vi "Autonomous Independent.vi"() -> ()   [LabVIEW 2015]
doc: "This VI is called when autonomous begins, and will automatically be terminated when autonomous ends. You can carry out timed or sensor driven robot movement independently without needing to return to the caller."
uses:
  <vilib>/Rock Robotics/WPI/Utilities/WPI_GetSetVariantRefNum.vi
  <vilib>/Rock Robotics/Network Tables/NT Read String.vi
  <vilib>/Rock Robotics/WPI/RobotDrive/WPI_RobotDriveArcadeDrive_Standard(NoSaturation).vi
  <vilib>/Rock Robotics/Network Tables/NT Write Numeric Array.vi
  Robot Global Data.vi
  <vilib>/Rock Robotics/Network Tables/NT Read Number.vi
  <vilib>/Rock Robotics/WPI/Solenoid/WPI_SolenoidSetEnum.vi
  <vilib>/Rock Robotics/WPI/Solenoid/WPI_SolenoidValue.ctl
  <vilib>/Rock Robotics/WPI/Relay/WPI_RelayValue.ctl
panel:
  out "Current Movement, for debugging":T1 {"Y Joystick Value" scale=1.0..-1.0; "X Joystick Value" scale=-1.0..1.0}
  in  "Array of robot movements":T2(array[cluster])=[{"X Joystick Value"=0.39393939393939403, "Y Joystick Value"=0.0, "Delay (sec)"=1.0, "Movement Name"="turn"}, {"X Joystick Value"=-0.3737373737373737, "Y Joystick Value"=0.0, "Delay (sec)"=1.0, "Movement Name"="turn back"}] {"Y Joystick Value" scale=1.0..-1.0; "X Joystick Value" scale=-1.0..1.0}
  # "Be sure to right-click and choose Data Operations>>Make Current Value default if you want to save the array values with the VI"
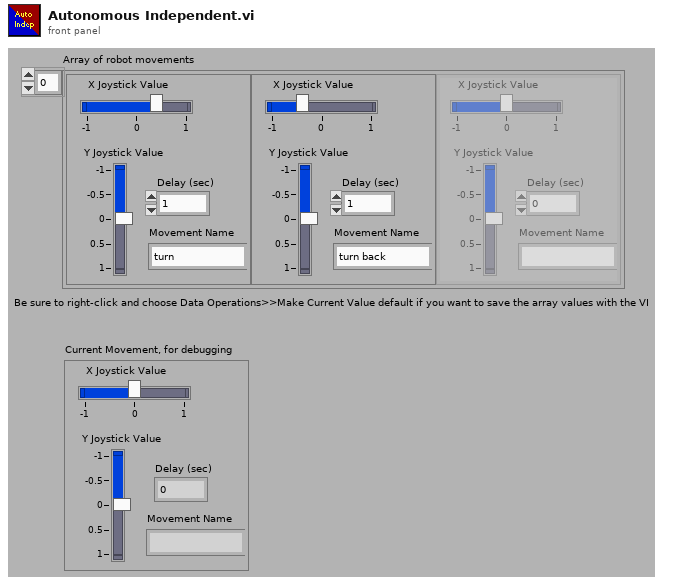
[diagram p1: front panel]
types:
  T1 = cluster{"X Joystick Value":dbl, "Y Joystick Value":dbl, "Delay (sec)":dbl, "Movement Name":string}
  T2 = cluster{"X Joystick Value":dbl, "Y Joystick Value":dbl, "Delay (sec)":dbl, "Movement Name":string}[]
  T3 = typedef "WPI_JoystickDevRef.ctl" = cluster{"Device":T4}
  T4 = typedef "WPI_JoystickDeviceEnum.ctl" = enum16{"USB 0", "USB 1", "USB 2", "USB 3", "USB 4", "USB 5"}
  T5 = typedef "WPI_RelayValue.ctl" = enum16{"Off", "On", "Forward", "Reverse"}
  T6 = typedef "WPI_SolenoidValue.ctl" = enum16{"Off", "On", "Forward", "Reverse"}
  T7 = typedef "WPI_RobotDriveDevRef.ctl" = cluster{"DevStatus":errorcluster, "Motors[]":T8[], "Square Inputs":bool, "Max Output":dbl}
  T8 = typedef "WPI_MotorControlDeviceRef.ctl" = cluster{"DeviceStatus":errorcluster, "Type":T9, "PWM":cluster{"PWM Channel":T10, "DeadBand":T11}, "CAN":cluster{"Device Number":u8, "Control Mode":T12, "Semaphore":T13, "Max Vout":dbl, "TalonSRX Control Mode":T14}, "Invert":bool}
  T9 = typedef "WPI_MotorControlType.ctl" = enum16{"PWM", "CAN", "CANTalonSRX"}
  T10 = typedef "FPGA_DIOPWMChannel.ctl" = enum8{"PWM 0", "PWM 1", "PWM 2", "PWM 3", "PWM 4", "PWM 5", "PWM 6", "PWM 7", "PWM 8", "PWM 9", "PWM MXP 0", "PWM MXP 1", "PWM MXP 2", "PWM MXP 3", "PWM MXP 4", "PWM MXP 5", "PWM MXP 6", "PWM MXP 7", "PWM MXP 8", "PWM MXP 9", "Invalid"}
  T11 = typedef "WPI_PWMDeadband.ctl" = cluster{"Name":string, "maxPositivePwm":i32, "minPositivePwm":i32, "centerPwm":i32, "maxNegativePwm":i32, "minNegativePwm":i32, "angularRange":u16}
  T12 = typedef "WPI_CANJaguar_ControlMode.ctl" = enum8{"Percent VBus", "Current", "Speed", "Position", "Voltage"}
  T13 = typedef "Semaphore RefNum" = refnum<k1>
  T14 = typedef "WPI_CANTalonSRX_APIControlMode.ctl" = enum8{"Percent VBus", "Speed", "Position", "Slave", "Unchanged / Invalid", "Voltage Compensation", "Current", "Motion Profile"}
  T15 = typedef "WPI_RelayDevRef.ctl" = cluster{"DevStatus":errorcluster, "Relay Channel":T16, "Relay Direction":T17}
  T16 = typedef "FPGA_DIORelayChannel.ctl" = enum8{"Relay 0", "Relay 1", "Relay 2", "Relay 3", "Invalid"}
  T17 = typedef "WPI_RelayDirection.ctl" = enum16{"Both directions", "Forward only", "Reverse only"}
  T18 = typedef "WPI_SolenoidDevRef.ctl" = cluster{"DevStatus":errorcluster, "Pneumatics Control Module":u8, "Forward Solenoid Channel":T19, "Reverse Solenoid Channel":T19}
  T19 = typedef "WPI_SolenoidChannel.ctl" = enum8{"Solenoid 0", "Solenoid 1", "Solenoid 2", "Solenoid 3", "Solenoid 4", "Solenoid 5", "Solenoid 6", "Solenoid 7", "Invalid"}
  T20 = cluster{"Distance (ft)":dbl, "Center":cluster{dbl, dbl}, "Normalized Rect":cluster{"Numeric":dbl, "Numeric 2":dbl, "Numeric 3":dbl, "Numeric 5":dbl}}[]
  T21 = cluster{"Distance (ft)":dbl, "Center":cluster{dbl, dbl}, "Normalized Rect":cluster{"Numeric":dbl, "Numeric 2":dbl, "Numeric 3":dbl, "Numeric 5":dbl}}
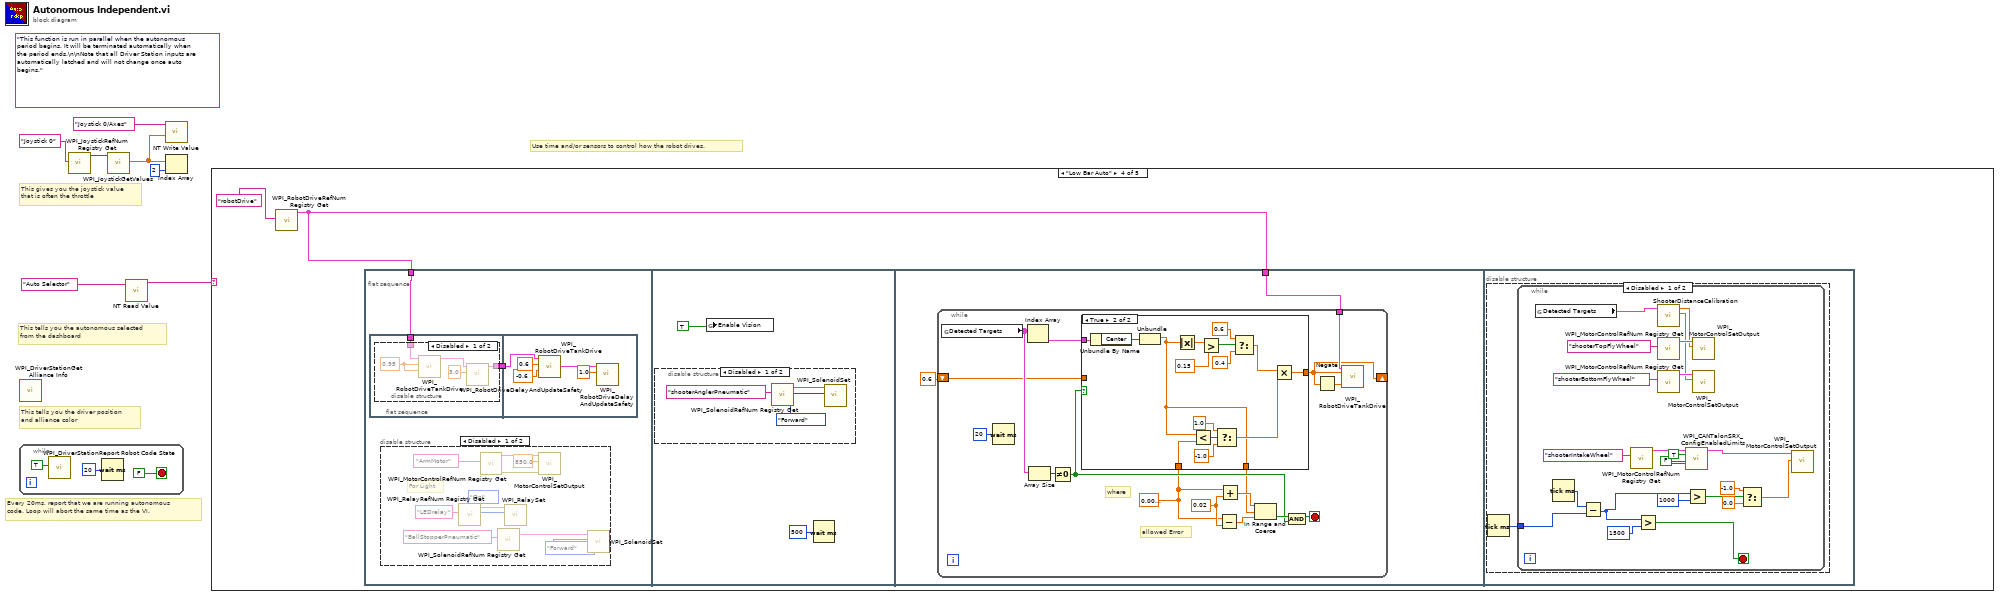
[diagram p0: block diagram]
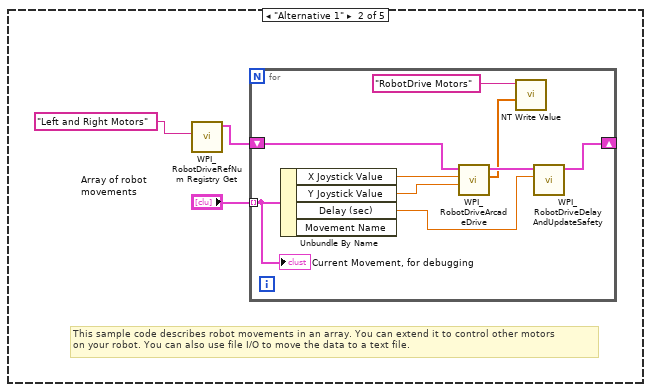
[diagram p3: hidden frame]
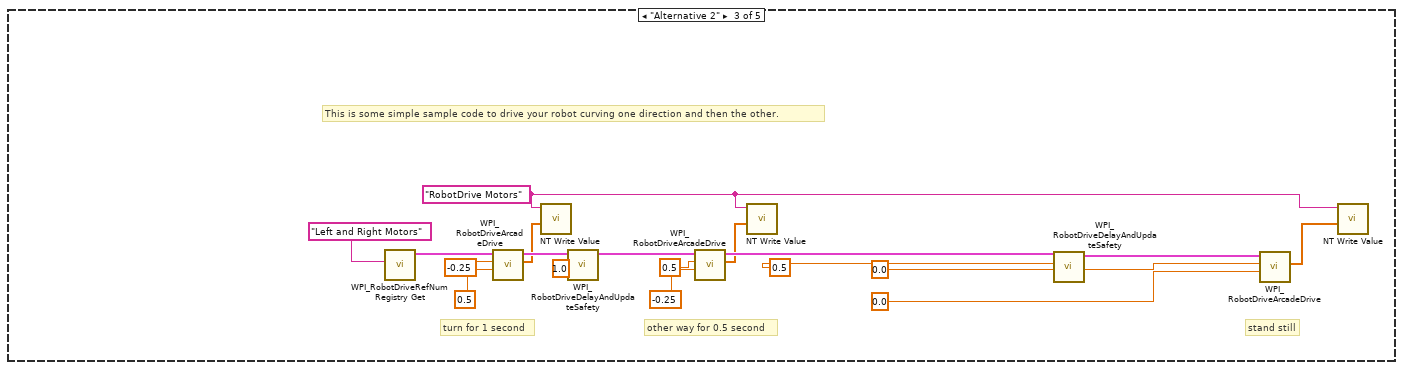
[diagram p4: hidden frame]
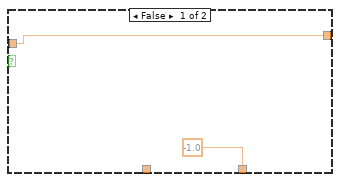
[diagram p8: hidden frame]
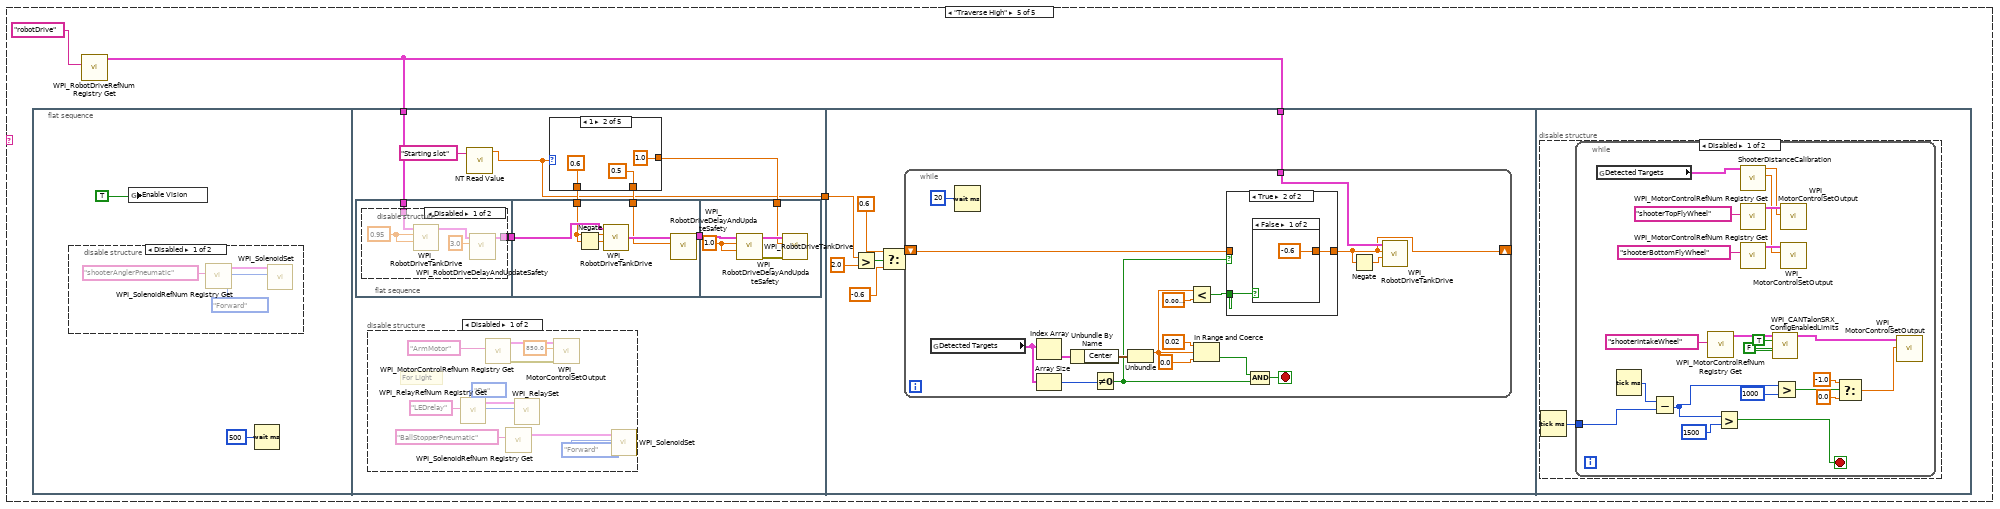
[diagram p10: hidden frame]
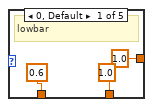
[diagram p12: hidden frame]
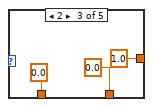
[diagram p13: hidden frame]
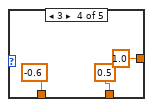
[diagram p14: hidden frame]
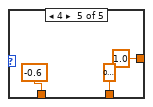
[diagram p15: hidden frame]
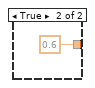
[diagram p19: hidden frame]
diagram:
  (unwired) "This function is run in parallel when the autonomous period begins. It will be terminated automatically when the period ends.\n\nNote that all Driver Station inputs are automatically latched and will not change once auto begins."
  # "This tells you the autonomous selected\nfrom the dashboard"
  # "Every 20ms, report that we are running autonomous\ncode. Loop will abort the same time as the VI."
  # "This gives you the joystick value\nthat is often the throttle"
  # "Use time and/or sensors to control how the robot drives."
  # "This tells you the driver position\nand alliance color"
  n1 = while {
    stop <- FALSE stop-if-true
    n2 = call <vilib>:"WPI_DriverStationReport Robot Code State.vi"("Autonomous"=TRUE) -> ()  [unwired: 10 in, 1 out]
    n3 = Wait (ms)(milliseconds to wait=u32 20) -> ()  [unwired: 1 out]
  }
  n4 = call <vilib>:"WPI_DriverStationGet Alliance Info.vi"() -> ()  [unwired: 12 out]
  n5 = call <vilib>:"WPI_JoystickRefNum Registry Get.vi"("refnum name"="Joystick 0") -> ("JoystickDevRef"=w6:T3)  [unwired: 1 in, 9 out]
  n6 = call <vilib>:"WPI_JoystickGetValues.vi"("JoystickDevRef"=w6) -> ("Axes"=w3:dbl[])  [unwired: 6 in, 4 out]
  n7 = call-poly <vilib>:"NT Read Value.vi"("Name"="Auto Selector") -> ("String"=w1:string)  [unwired: 9 in, 1 out]
  n8 = call-poly <vilib>:"NT Write Value.vi"("Numeric Array"=w3, "Name"="Joystick 0/Axes") -> ()  [unwired: 9 in, 1 out]
  n9 = Index Array(array=w3, index=2) -> ()  [unwired: 1 out]
  n10 = case shown="\"Low Bar Auto\"" w1 {
    frame "Nothing", Default {
      # "You can put your main auto here, or you can right-click on the case and make any\nother frame be the default case."
      # "This is the frame that will execute if no selection is made, or if it is not recognized"
    }
    frame "Alternative 1" {
      # "This sample code describes robot movements in an array. You can extend it to control other motors\non your robot. You can also use file I/O to move the data to a text file."
      n11 = call <vilib>:"WPI_RobotDriveRefNum Registry Get.vi"("refnum name"="Left and Right Motors") -> ("RobotDriveDevRef"=w12:T7)  [unwired: 1 in, 9 out]
      n12 = for {
        shift-right: [w20] -> _
        shift-left: w12 -> [w21]
        tunnel: "Array of robot movements" -> [w16] mode=indexing
        n13 = Unbundle By Name(w16) -> ("X Joystick Value"=w19:dbl, "Y Joystick Value"=w18:dbl, "Delay (sec)"=w17:dbl)  [unwired: 1 out]
        n14 = call-poly <vilib>:"WPI_RobotDriveArcadeDrive.vi"("Y axis value"=w18, "X axis value"=w19, "RobotDriveDevRef"=w21) -> ("Motor Values"=w14:dbl[], "RobotDriveDevRef"=w22:T7)  [unwired: 1 in, 6 out]
        n15 = call-poly <vilib>:"NT Write Value.vi"("Numeric Array"=w14, "Name"="RobotDrive Motors") -> ()  [unwired: 9 in, 1 out]
        n16 = call <vilib>:"WPI_RobotDriveDelayAndUpdateSafety.vi"("Delay (s)"=w17, "RobotDriveDevRef"=w22) -> ("RobotDriveDevRef 2"=w20:T7)  [unwired: 8 in, 1 out]
        "Current Movement, for debugging" <- w16
      }
    }
    frame "Alternative 2" {
      w24 = "RobotDrive Motors" ("Name")
      # "This is some simple sample code to drive your robot curving one direction and then the other."
      # "stand still"
      # "other way for 0.5 second"
      # "turn for 1 second"
      n17 = call <vilib>:"WPI_RobotDriveRefNum Registry Get.vi"("refnum name"="Left and Right Motors") -> ("RobotDriveDevRef"=w40:T7)  [unwired: 1 in, 9 out]
      n18 = call-poly <vilib>:"WPI_RobotDriveArcadeDrive.vi"("Y axis value"=0.5 ("X axis value"), "X axis value"=-0.25, "RobotDriveDevRef"=w40) -> ("Motor Values"=w23:dbl[], "RobotDriveDevRef"=w33:T7)  [unwired: 1 in, 6 out]
      n19 = call-poly <vilib>:"NT Write Value.vi"("Numeric Array"=w23, "Name"=w24) -> ()  [unwired: 9 in, 1 out]
      n20 = call <vilib>:"WPI_RobotDriveDelayAndUpdateSafety.vi"("Delay (s)"=1.0, "RobotDriveDevRef"=w33) -> ("RobotDriveDevRef 2"=w34:T7)  [unwired: 8 in, 1 out]
      n21 = call-poly <vilib>:"WPI_RobotDriveArcadeDrive.vi"("Y axis value"=-0.25 ("X axis value"), "X axis value"=0.5, "RobotDriveDevRef"=w34) -> ("Motor Values"=w25:dbl[], "RobotDriveDevRef"=w35:T7)  [unwired: 1 in, 6 out]
      n22 = call-poly <vilib>:"NT Write Value.vi"("Numeric Array"=w25, "Name"=w24) -> ()  [unwired: 9 in, 1 out]
      n23 = call <vilib>:"WPI_RobotDriveDelayAndUpdateSafety.vi"("Delay (s)"=0.5, "RobotDriveDevRef"=w35) -> ("RobotDriveDevRef 2"=w36:T7)  [unwired: 8 in, 1 out]
      n24 = call-poly <vilib>:"WPI_RobotDriveArcadeDrive.vi"("Y axis value"=0.0 ("X axis value"), "X axis value"=0.0, "RobotDriveDevRef"=w36) -> ("Motor Values"=w26:dbl[])  [unwired: 1 in, 7 out]
      n25 = call-poly <vilib>:"NT Write Value.vi"("Numeric Array"=w26, "Name"=w24) -> ()  [unwired: 9 in, 1 out]
    }
    frame "Low Bar Auto" {
      n26 = call <vilib>:"WPI_RobotDriveRefNum Registry Get.vi"("refnum name"="robotDrive") -> ("RobotDriveDevRef"=w41:T7)  [unwired: 9 in, 1 out]
      n27 = flat-sequence {
        tunnel: w41 -> [w44]
        tunnel: w41 -> [w73]
        frame #0 {
          n28 = flat-sequence {
            tunnel: w44 -> [w56]
            tunnel: [w55] -> w43
            tunnel: w43 -> [w63]
            frame #0 {
              n29 = disable-structure shown="Disabled" {
                disable-tunnel: w56 -> [w59 w62]
                disable-tunnel: [w58 w62] -> w55
                frame Disabled {
                  w57 = 0.95 ("Left axis value")
                  n30 = call <vilib>:"WPI_RobotDriveTankDrive.vi"("Right axis value"=w57, "Left axis value"=w57, "RobotDriveDevRef"=w59) -> ("RobotDriveDevRef"=w60:T7)  [unwired: 6 in, 2 out]
                  n31 = call <vilib>:"WPI_RobotDriveDelayAndUpdateSafety.vi"("Delay (s)"=3.0, "RobotDriveDevRef"=w60) -> ("RobotDriveDevRef 2"=w58:T7)  [unwired: 8 in, 1 out]
                }
                frame Enabled {
                }
              }
            }
            frame #1 {
              n32 = call <vilib>:"WPI_RobotDriveTankDrive.vi"("Right axis value"=-0.6, "Left axis value"=0.6, "RobotDriveDevRef"=w63) -> ("RobotDriveDevRef"=w66:T7)  [unwired: 6 in, 2 out]
              n33 = call <vilib>:"WPI_RobotDriveDelayAndUpdateSafety.vi"("Delay (s)"=1.0, "RobotDriveDevRef"=w66) -> ()  [unwired: 8 in, 2 out]
            }
          }
          n34 = disable-structure shown="Disabled" {
            frame Disabled {
              # "For Light"
              n35 = call <vilib>:"WPI_RelayRefNum Registry Get.vi"("refnum name"="LEDrelay") -> ("RelayDevRef"=w46:T15)  [unwired: 9 in, 1 out]
              n36 = call <vilib>:"WPI_MotorControlRefNum Registry Get.vi"("refnum name"="ArmMotor") -> ("error out"=w51:errorcluster, "MotorControlDevRef"=w49:T8)  [unwired: 9 in]
              n37 = call <vilib>:"WPI_SolenoidRefNum Registry Get.vi"("refnum name"="BallStopperPneumatic") -> ("SolenoidDevRef"=w52:T18)  [unwired: 9 in, 1 out]
              n38 = call <vilib>:"WPI_RelaySet.vi"("RelayValue"=WPI_RelayValue."On", "RelayDevRef"=w46) -> ()  [unwired: 8 in, 2 out]
              n39 = call <vilib>:"WPI_MotorControlSetOutput.vi"("error in (no error)"=w51, "Output"=850.0, "MotorControlDevRef"=w49) -> ()  [unwired: 6 in, 3 out]
              n40 = call-poly <vilib>:"WPI_SolenoidSet.vi"("Value"=WPI_SolenoidValue."Forward", "SolenoidDevRef"=w52) -> ()  [unwired: 8 in, 2 out]
            }
            frame Enabled {
            }
          }
        }
        frame #1 {
          n41 = disable-structure shown="Disabled" {
            frame Disabled {
              n42 = call <vilib>:"WPI_SolenoidRefNum Registry Get.vi"("refnum name"="shooterAnglerPneumatic") -> ("SolenoidDevRef"=w71:T18)  [unwired: 9 in, 1 out]
              n43 = call-poly <vilib>:"WPI_SolenoidSet.vi"("Value"=WPI_SolenoidValue."Forward", "SolenoidDevRef"=w71) -> ()  [unwired: 8 in, 2 out]
            }
            frame Enabled {
            }
          }
          n44 = global write "Robot Global Data.vi" "Enable Vision"(TRUE ("Enable Vision")) -> ()
          n45 = Wait (ms)(milliseconds to wait=u32 500) -> ()  [unwired: 1 out]
        }
        frame #2 {
          n46 = while {
            tunnel: w73 -> [w88]
            shift-right: [w77] -> _
            shift-left: 0.6 ("t") -> [w78]
            stop <- w87 stop-if-true
            w75 = 0.009999999999999997 ("x")
            w80 = 0.02
            # "allowed Error"
            # "where"
            n47 = global read "Robot Global Data.vi" "Detected Targets"() -> (w86:T20)
            n48 = Wait (ms)(milliseconds to wait=u32 20) -> ()  [unwired: 1 out]
            n49 = Index Array(array=w86) -> (element=w90:T21)  [unwired: 1 in]
            n50 = Array Size(array=w86) -> (size(s)=w85:i32)
            n51 = Not Equal To 0?(x=w85) -> (x != 0?=w79:bool)
            n52 = case shown="True" w79 {
              tunnel: w90 -> [_ w107]
              tunnel: w75 -> [_ w105]
              tunnel: [w92 w94] -> w77
              tunnel: w78 -> [w92 _]
              tunnel: [-1.0 ("x") w93] -> w76
              frame False {
              }
              frame True {
                n53 = Unbundle By Name(w107) -> ("Center"=w106:cluster{dbl, dbl})
                n54 = Unbundle(w106) -> (w93:dbl)  [unwired: 1 out]
                n55 = Absolute Value(x=w93) -> (abs(x)=w104:dbl)
                n56 = Less?(x=w93, y=w105) -> (x < y?=w99:bool)
                n57 = Greater?(x=w104, y=0.15) -> (0:w102:bool)
                n58 = Select(t=1.0, s=w99, f=-1.0) -> (s? t:f=w95:dbl)
                n59 = Select(t=0.6, s=w102, f=0.4) -> (s? t:f=w96:dbl)
                n60 = Multiply(x=w96, y=w95) -> (x*y=w94:dbl)
              }
            }
            n61 = Subtract(x=w75, y=w80) -> (x-y=w81:dbl)
            n62 = Add(x=w75, y=w80) -> (x+y=w82:dbl)
            n63 = In Range and Coerce(upper limit=w82, x=w76, lower limit=w81) -> (In Range?=w89:bool)  [unwired: 1 out]
            n64 = Compound Arithmetic op=AND(w89, w79) -> (w87:bool)
            n65 = Negate(x=w77) -> (-x=w83:dbl)
            n66 = call <vilib>:"WPI_RobotDriveTankDrive.vi"("Right axis value"=w83, "Left axis value"=w77, "RobotDriveDevRef"=w88) -> ()  [unwired: 6 in, 3 out]
          }
        }
        frame #3 {
          n67 = disable-structure shown="Disabled" {
            frame Disabled {
              n68 = Tick Count (ms)() -> (millisecond timer value=w108:u32)
              n69 = while {
                tunnel: w108 -> [w128]
                stop <- w126 stop-if-true
                w109 = FALSE ("Forward Limit Switch Enable")
                n70 = global read "Robot Global Data.vi" "Detected Targets"() -> (w121:T20)
                n71 = Tick Count (ms)() -> (millisecond timer value=w129:u32)
                n72 = Subtract(x=w129, y=w128) -> (x-y=w120:u32)
                n73 = call <vilib>:"WPI_MotorControlRefNum Registry Get.vi"("refnum name"="shooterIntakeWheel") -> ("MotorControlDevRef"=w112:T8)  [unwired: 9 in, 1 out]
                n74 = Greater?(x=w120, y=u32 1500) -> (0:w126:bool)
                n75 = call "ShooterDistanceCalibration.vi"("Detected Totes"=w121) -> ("bottomFlyWheelConstant"=w122:dbl, "TopFlyWheelConstant"=w123:dbl)  [unwired: 9 in]
                n76 = call <vilib>:"WPI_MotorControlRefNum Registry Get.vi"("refnum name"="shooterTopFlyWheel") -> ("MotorControlDevRef"=w124:T8)  [unwired: 9 in, 1 out]
                n77 = call <vilib>:"WPI_MotorControlRefNum Registry Get.vi"("refnum name"="shooterBottomFlyWheel") -> ("MotorControlDevRef"=w125:T8)  [unwired: 9 in, 1 out]
                n78 = call <vilib>:"WPI_CANTalonSRX_ConfigEnabledLimits.vi"("CAN Talon SRX Ref"=w112, "Override Limit Switches"=TRUE, "Forward Limit Switch Enable"=w109, "Reverse Limit Switch Enable"=w109) -> ("CAN Talon SRX Ref"=w111:T8)  [unwired: 10 in, 1 out]
                n79 = Greater?(x=w120, y=u32 1000) -> (0:w118:bool)
                n80 = call <vilib>:"WPI_MotorControlSetOutput.vi"("Output"=w123, "MotorControlDevRef"=w124) -> ()  [unwired: 7 in, 3 out]
                n81 = call <vilib>:"WPI_MotorControlSetOutput.vi"("Output"=w122, "MotorControlDevRef"=w125) -> ()  [unwired: 7 in, 3 out]
                n82 = Select(t=-1.0, s=w118, f=0.0) -> (s? t:f=w115:dbl)
                n83 = call <vilib>:"WPI_MotorControlSetOutput.vi"("Output"=w115, "MotorControlDevRef"=w111) -> ()  [unwired: 7 in, 3 out]
              }
            }
            frame Enabled {
            }
          }
        }
      }
    }
    frame "Traverse High" {
      n84 = flat-sequence {
        tunnel: w132 -> [w145]
        tunnel: [w139] -> w131
        tunnel: w132 -> [w197]
        tunnel: w131 -> [w192]
        frame #0 {
          n85 = disable-structure shown="Disabled" {
            frame Disabled {
              n86 = call <vilib>:"WPI_SolenoidRefNum Registry Get.vi"("refnum name"="shooterAnglerPneumatic") -> ("SolenoidDevRef"=w137:T18)  [unwired: 9 in, 1 out]
              n87 = call-poly <vilib>:"WPI_SolenoidSet.vi"("Value"=WPI_SolenoidValue."Forward", "SolenoidDevRef"=w137) -> ()  [unwired: 8 in, 2 out]
            }
            frame Enabled {
            }
          }
          n88 = global write "Robot Global Data.vi" "Enable Vision"(TRUE ("Enable Vision")) -> ()
          n89 = Wait (ms)(milliseconds to wait=u32 500) -> ()  [unwired: 1 out]
        }
        frame #1 {
          n90 = flat-sequence {
            tunnel: w145 -> [w173]
            tunnel: [w172] -> w146
            tunnel: w146 -> [w184]
            tunnel: w143 -> [w183]
            tunnel: w142 -> [w181]
            tunnel: [w180] -> w141
            tunnel: w141 -> [w190]
            tunnel: w140 -> [w186]
            frame #0 {
              n91 = disable-structure shown="Disabled" {
                disable-tunnel: w173 -> [w176 w179]
                disable-tunnel: [w175 w179] -> w172
                frame Disabled {
                  w174 = 0.95 ("Left axis value")
                  n92 = call <vilib>:"WPI_RobotDriveTankDrive.vi"("Right axis value"=w174, "Left axis value"=w174, "RobotDriveDevRef"=w176) -> ("RobotDriveDevRef"=w177:T7)  [unwired: 6 in, 2 out]
                  n93 = call <vilib>:"WPI_RobotDriveDelayAndUpdateSafety.vi"("Delay (s)"=3.0, "RobotDriveDevRef"=w177) -> ("RobotDriveDevRef 2"=w175:T7)  [unwired: 8 in, 1 out]
                }
                frame Enabled {
                }
              }
            }
            frame #1 {
              n94 = Negate(x=w183) -> (-x=w182:dbl)
              n95 = call <vilib>:"WPI_RobotDriveTankDrive.vi"("Right axis value"=w182, "Left axis value"=w183, "RobotDriveDevRef"=w184) -> ("RobotDriveDevRef"=w185:T7)  [unwired: 6 in, 2 out]
              n96 = call <vilib>:"WPI_RobotDriveDelayAndUpdateSafety.vi"("Delay (s)"=w181, "RobotDriveDevRef"=w185) -> ("RobotDriveDevRef 2"=w180:T7)  [unwired: 8 in, 1 out]
            }
            frame #2 {
              w189 = 1.0 ("Left axis value")
              n97 = call <vilib>:"WPI_RobotDriveTankDrive.vi"("Right axis value"=w189, "Left axis value"=w189, "RobotDriveDevRef"=w190) -> ("error out"=w188:errorcluster, "RobotDriveDevRef"=w187:T7)  [unwired: 6 in, 1 out]
              n98 = call <vilib>:"WPI_RobotDriveDelayAndUpdateSafety.vi"("error in (no error)"=w188, "Delay (s)"=w186, "RobotDriveDevRef"=w187) -> ()  [unwired: 7 in, 2 out]
            }
          }
          n99 = disable-structure shown="Disabled" {
            frame Disabled {
              # "For Light"
              n100 = call <vilib>:"WPI_RelayRefNum Registry Get.vi"("refnum name"="LEDrelay") -> ("RelayDevRef"=w163:T15)  [unwired: 9 in, 1 out]
              n101 = call <vilib>:"WPI_MotorControlRefNum Registry Get.vi"("refnum name"="ArmMotor") -> ("error out"=w168:errorcluster, "MotorControlDevRef"=w166:T8)  [unwired: 9 in]
              n102 = call <vilib>:"WPI_SolenoidRefNum Registry Get.vi"("refnum name"="BallStopperPneumatic") -> ("SolenoidDevRef"=w169:T18)  [unwired: 9 in, 1 out]
              n103 = call <vilib>:"WPI_RelaySet.vi"("RelayValue"=WPI_RelayValue."On", "RelayDevRef"=w163) -> ()  [unwired: 8 in, 2 out]
              n104 = call <vilib>:"WPI_MotorControlSetOutput.vi"("error in (no error)"=w168, "Output"=850.0, "MotorControlDevRef"=w166) -> ()  [unwired: 6 in, 3 out]
              n105 = call-poly <vilib>:"WPI_SolenoidSet.vi"("Value"=WPI_SolenoidValue."Forward", "SolenoidDevRef"=w169) -> ()  [unwired: 8 in, 2 out]
            }
            frame Enabled {
            }
          }
          n106 = call-poly <vilib>:"NT Read Value.vi"("Name"="Starting slot") -> ("Numeric"=w139:dbl)  [unwired: 9 in, 1 out]
          n107 = case shown="1" w139 {
            tunnel: [0.6 ("Left axis value") 0.6 ("Left axis value") 0.0 ("Left axis value") -0.6 ("Left axis value") -0.6 ("Left axis value")] -> w143
            tunnel: [1.0 ("Left axis value") 0.5 ("Delay (s)") 0.0 ("Delay (s)") 0.5 ("Left axis value") 0.9999999999999999 ("Left axis value")] -> w142
            tunnel: [1.0 ("Left axis value") 1.0 ("Left axis value") 1.0 ("Left axis value") 1.0 ("Left axis value") 1.0 ("Left axis value")] -> w140
            frame 0, Default {
              # "lowbar"
            }
            frame 1 {
            }
            frame 2 {
            }
            frame 3 {
            }
            frame 4 {
            }
          }
        }
        frame #2 {
          n108 = Greater?(x=w192, y=2.0) -> (0:w193:bool)
          n109 = Select(t=0.6 ("Left axis value"), s=w193, f=-0.6) -> (s? t:f=w195:dbl)
          n110 = while {
            tunnel: w197 -> [w209]
            shift-right: [w200] -> _
            shift-left: w195 -> [w198]
            stop <- w208 stop-if-true
            n111 = global read "Robot Global Data.vi" "Detected Targets"() -> (w207:T20)
            n112 = Wait (ms)(milliseconds to wait=u32 20) -> ()  [unwired: 1 out]
            n113 = Index Array(array=w207) -> (element=w214:T21)  [unwired: 1 in]
            n114 = Array Size(array=w207) -> (size(s)=w206:i32)
            n115 = Unbundle By Name(w214) -> ("Center"=w213:cluster{dbl, dbl})
            n116 = Not Equal To 0?(x=w206) -> (x != 0?=w199:bool)
            n117 = Unbundle(w213) -> (w204:dbl)  [unwired: 1 out]
            n118 = Less?(x=w204, y=0.009999999999999997 ("x")) -> (x < y?=w201:bool)
            n119 = In Range and Coerce(upper limit=0.02, x=w204, lower limit=0.0) -> (In Range?=w210:bool)  [unwired: 1 out]
            n120 = case shown="True" w199 {
              tunnel: w201 -> [_ w217]
              tunnel: [w215 w216] -> w200
              tunnel: w198 -> [w215 _]
              frame False {
              }
              frame True {
                n121 = case shown="False" w217 {
                  tunnel: [-0.6 ("Left axis value") 0.6 ("Left axis value")] -> w216
                  frame False {
                  }
                  frame True {
                  }
                }
              }
            }
            n122 = Compound Arithmetic op=AND(w210, w199) -> (w208:bool)
            n123 = Negate(x=w200) -> (-x=w202:dbl)
            n124 = call <vilib>:"WPI_RobotDriveTankDrive.vi"("Right axis value"=w202, "Left axis value"=w200, "RobotDriveDevRef"=w209) -> ()  [unwired: 6 in, 3 out]
          }
        }
        frame #3 {
          n125 = disable-structure shown="Disabled" {
            frame Disabled {
              n126 = Tick Count (ms)() -> (millisecond timer value=w220:u32)
              n127 = while {
                tunnel: w220 -> [w240]
                stop <- w238 stop-if-true
                w221 = FALSE ("Forward Limit Switch Enable")
                n128 = global read "Robot Global Data.vi" "Detected Targets"() -> (w233:T20)
                n129 = Tick Count (ms)() -> (millisecond timer value=w241:u32)
                n130 = Subtract(x=w241, y=w240) -> (x-y=w232:u32)
                n131 = call <vilib>:"WPI_MotorControlRefNum Registry Get.vi"("refnum name"="shooterIntakeWheel") -> ("MotorControlDevRef"=w224:T8)  [unwired: 9 in, 1 out]
                n132 = Greater?(x=w232, y=u32 1500) -> (0:w238:bool)
                n133 = call "ShooterDistanceCalibration.vi"("Detected Totes"=w233) -> ("bottomFlyWheelConstant"=w234:dbl, "TopFlyWheelConstant"=w235:dbl)  [unwired: 9 in]
                n134 = call <vilib>:"WPI_MotorControlRefNum Registry Get.vi"("refnum name"="shooterTopFlyWheel") -> ("MotorControlDevRef"=w236:T8)  [unwired: 9 in, 1 out]
                n135 = call <vilib>:"WPI_MotorControlRefNum Registry Get.vi"("refnum name"="shooterBottomFlyWheel") -> ("MotorControlDevRef"=w237:T8)  [unwired: 9 in, 1 out]
                n136 = call <vilib>:"WPI_CANTalonSRX_ConfigEnabledLimits.vi"("CAN Talon SRX Ref"=w224, "Override Limit Switches"=TRUE, "Forward Limit Switch Enable"=w221, "Reverse Limit Switch Enable"=w221) -> ("CAN Talon SRX Ref"=w223:T8)  [unwired: 10 in, 1 out]
                n137 = Greater?(x=w232, y=u32 1000) -> (0:w230:bool)
                n138 = call <vilib>:"WPI_MotorControlSetOutput.vi"("Output"=w235, "MotorControlDevRef"=w236) -> ()  [unwired: 7 in, 3 out]
                n139 = call <vilib>:"WPI_MotorControlSetOutput.vi"("Output"=w234, "MotorControlDevRef"=w237) -> ()  [unwired: 7 in, 3 out]
                n140 = Select(t=-1.0, s=w230, f=0.0) -> (s? t:f=w227:dbl)
                n141 = call <vilib>:"WPI_MotorControlSetOutput.vi"("Output"=w227, "MotorControlDevRef"=w223) -> ()  [unwired: 7 in, 3 out]
              }
            }
            frame Enabled {
            }
          }
        }
      }
      n142 = call <vilib>:"WPI_RobotDriveRefNum Registry Get.vi"("refnum name"="robotDrive") -> ("RobotDriveDevRef"=w132:T7)  [unwired: 9 in, 1 out]
    }
  }
